vi "currentTreeItemPath.vi"(8 "error in":errorcluster, 11 "TreeRef":refnum<vi>) -> (0 "error out":errorcluster, 2 "treePath":string)   [LabVIEW 2013]
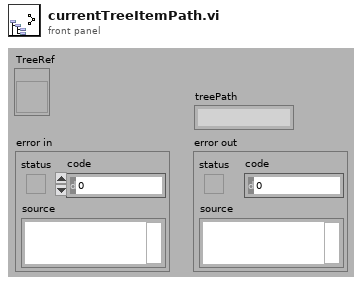
[diagram p1: front panel]
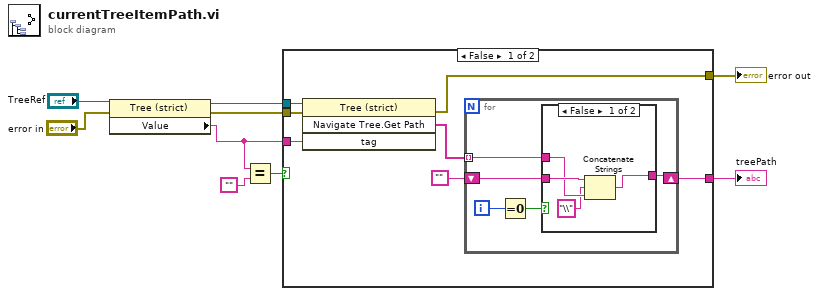
[diagram p0: block diagram]
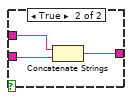
[diagram p2: hidden frame]
diagram:
  n1 = property class="Tree (strict)"(reference="TreeRef", error in="error in") -> (reference out=w8:refnum<vi>, error out=w7:errorcluster, "Value"=w3:string)
  n2 = Equal?(x=w3, y="") -> (x = y?=w1:bool)
  n3 = case shown="False" w1 {
    tunnel: w8 -> [w16 _]
    tunnel: w7 -> [w15 w29]
    tunnel: [w12 _] -> w5
    tunnel: [w11 w29] -> w4
    tunnel: w3 -> [w10 _]
    frame False {
      n4 = invoke class="Tree (strict)" method="Navigate Tree.Get Path"(reference=w16, error in=w15, "tag"=w10) -> (error out=w11:errorcluster, "Navigate Tree:Get Path"=w14:string[])  [unwired: 1 in, 2 out]
      n5 = for {
        tunnel: w14 -> [w18] mode=indexing
        shift-right: [w17] -> w12
        shift-left: "" -> [w19]
        i -> [w21]
        n6 = Equal To 0?(x=w21) -> (x = 0?=w20:bool)
        n7 = case shown="False" w20 {
          tunnel: w19 -> [w25 w28]
          tunnel: w18 -> [w24 w27]
          tunnel: [w22 w26] -> w17
          frame False {
            n8 = Concatenate Strings(w25, "\\" ("string"), w24) -> (w22:string)
          }
          frame True {
            n9 = Concatenate Strings(w27, w28) -> (w26:string)
          }
        }
      }
    }
    frame True {
      # "For some reason, feeding a \"\" caused Get Path node to return\n the path from the previous call"
    }
  }
  "treePath" <- w5
  "error out" <- w4
